vi "RunSet.vi"(8 "error in (no error)":errorcluster caption="错误输入（无错误）", 10 "TIMEBASE命令子系统":string(combo), 11 "VISA资源名称":refnum<visa-resource-name>) -> (0 "error out":errorcluster caption="错误输出", 3 "VISA资源名称 2":refnum<visa-resource-name>)   [LabVIEW 2018]
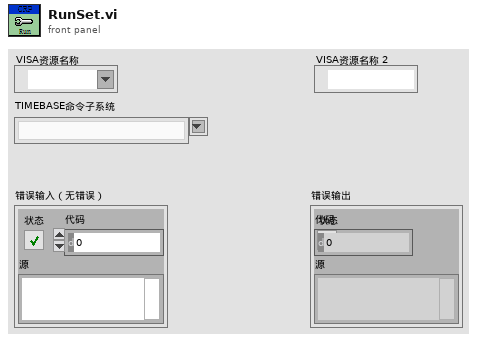
[diagram p1: front panel]
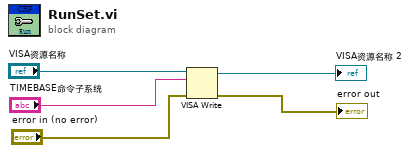
[diagram p0: block diagram]
diagram:
  n1 = VISA Write(VISA resource name="VISA资源名称", write buffer="TIMEBASE命令子系统", error in (no error)="error in (no error)") -> (VISA resource name out=→"VISA资源名称 2":refnum<visa-resource-name>, error out=→"error out":errorcluster)  [unwired: 1 out]
